vi "DeSerializeMethod.vi"(0 "object in":refnum<class "Serializer.lvclass">, 2 "String":string, 5 "error in (no error)":errorcluster) -> (14 "object out":refnum<class "Serializer.lvclass">, 15 "Class":string, 16 "Method":string, 17 "Inputsstring":string, 19 "error out":errorcluster)   [LabVIEW 2018, in "Serializer.lvclass"]
doc: "Deserialize the input string to the known format of Class, Method and Inputs"
uses:
  Serializer.lvclass
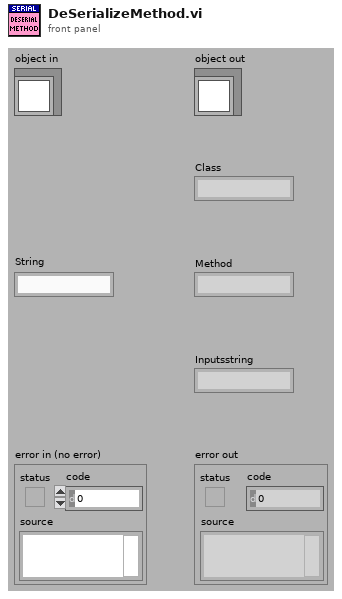
[diagram p1: front panel]
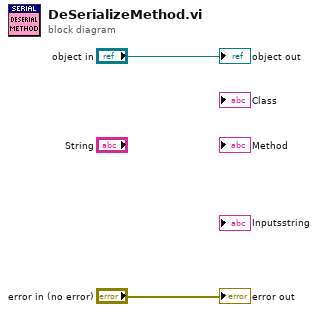
[diagram p0: block diagram]
diagram:
  "error out" <- "error in (no error)"
  "object out" <- "object in"
